vi "Module - RH_JONATHAN_LAMA.vi"() -> ()   [LabVIEW 2020]
uses:
  Control/State - eFGV.ctl
panel:
  out "Site Name":string="RH JONATHAN (13.65 kWp)"
  out "BANK-02-TEMP":dbl caption="T_bat" format="%#_g °C"
  out "BANK-02-IDC":dbl caption="I_bat" format="%#_g A"
  out "BANK-02-VDC":dbl caption="V_bat" format="%#_g V"
  out "BANK-02-SOC":dbl caption="SOC" format="%#_g %"
  out "PM-01-STATUS":bool
  out "SI-M-STATUS":bool
  out "BANK-01-TEMP":dbl caption="T_bat" format="%#_g °C"
  out "BANK-01-IDC":dbl caption="I_bat" format="%#_g A"
  out "BANK-01-VDC":dbl caption="V_bat" format="%#_g V"
  out "BANK-01-SOC":dbl caption="SOC" format="%#_g %"
  out "SB-02-STATUS":bool
  out "SB-02-B-IDC":dbl caption="B.Idc" format="%.0f A"
  out "SB-02-B-VDC":dbl caption="B.Vdc" format="%.0f V"
  out "SB-02-A-IDC":dbl caption="A.Idc" format="%.0f A"
  out "SB-02-A-VDC":dbl caption="A.Vdc" format="%.0f V"
  out "SB-02-PAC":dbl caption="Pac" format="%#_g W"
  out "SB-01-STATUS":bool
  out "SB-01-B-IDC":dbl caption="B.Idc" format="%.1f A"
  out "SB-01-B-VDC":dbl caption="B.Vdc" format="%.0f V"
  out "SB-01-A-IDC":dbl caption="A.Idc" format="%.1f A"
  out "SB-01-A-VDC":dbl caption="A.Vdc" format="%.0f V"
  out "SB-01-PAC":dbl caption="Pac" format="%.0f W"
  out "PM-01-FREQ":dbl caption="Freq" format="%.0f Hz"
  out "PM-01-IAC":dbl caption="Iac" format="%.0f A"
  out "PM-01-VAC":dbl caption="Vac" format="%.0f V"
  out "PM-01-PAC":dbl caption="Pac" format="%.0f W"
  out "SI-M-FREQ":dbl caption="FREQ" format="%.0f Hz"
  out "SI-M-L3":dbl caption="L3" format="%.0f V"
  out "SI-M-L2":dbl caption="L2" format="%.0f V"
  out "SI-M-L1":dbl caption="L1" format="%.0f V"
  out "SI-M-PAC":dbl caption="Pac" format="%.0f W"
  # "BANK-1"
  # "BANK-2"
  # "SI"
  # "PM-01"
  # "SB-02"
  # "SB-01"
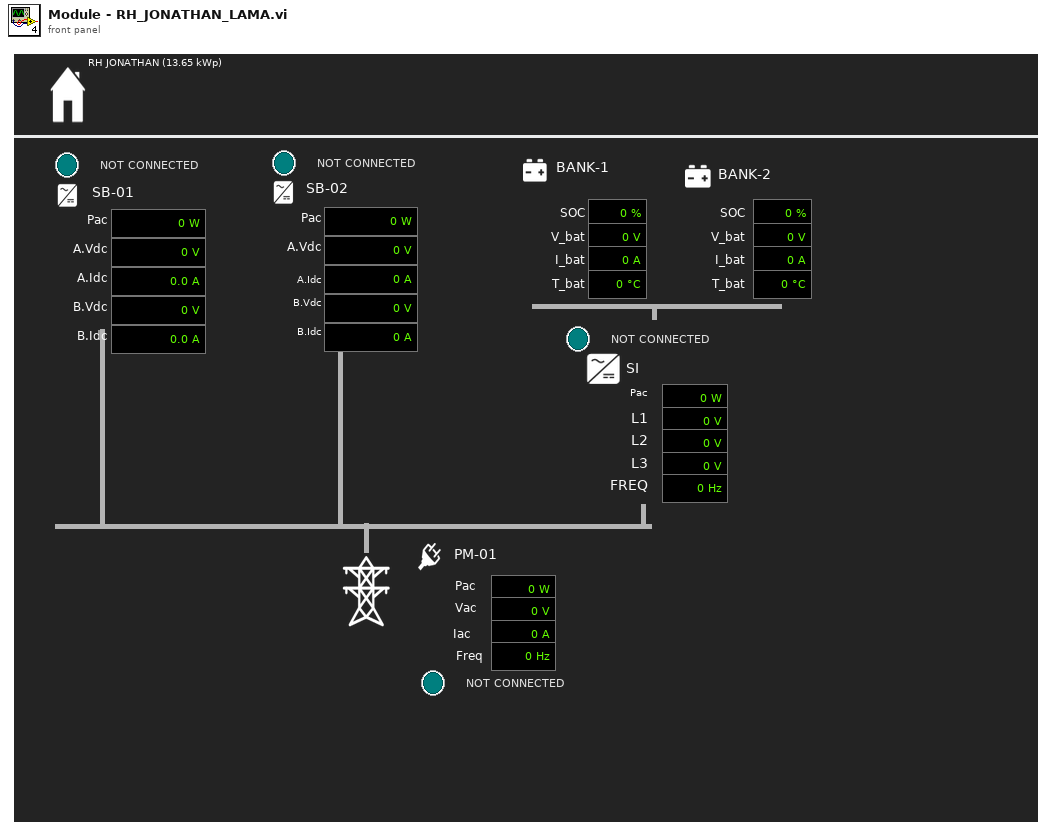
[diagram p1: front panel]
types:
  T1 = typedef "State - eFGV.ctl" = enum16{"Init", "Read", "Write", "Close"}
  T2 = typedef "Device Name.ctl" = enum16{"SB-01", "SB-02", "BANK-01", "BANK-02", "SI-M", "SI-S01", "SI-S02", "PM-01"}
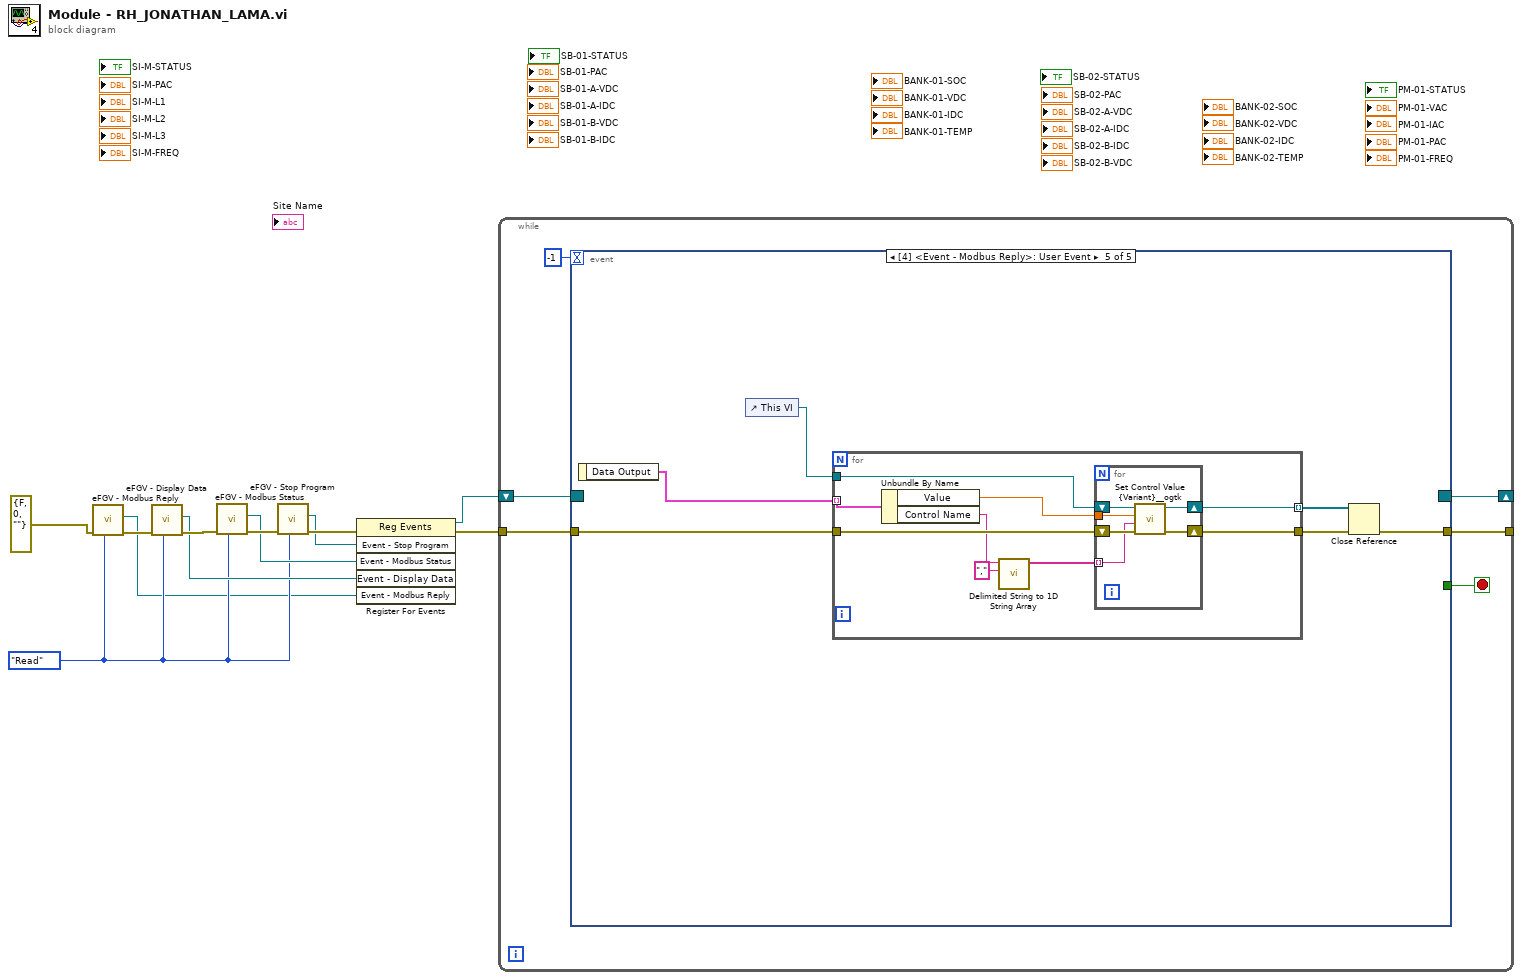
[diagram p0: block diagram]
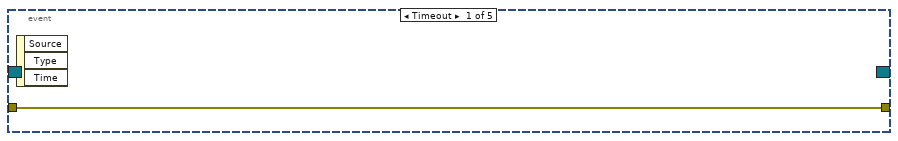
[diagram p2: hidden frame]
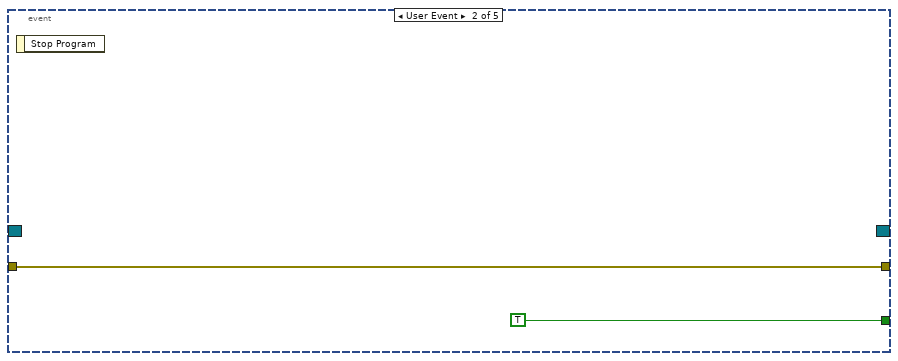
[diagram p3: hidden frame]
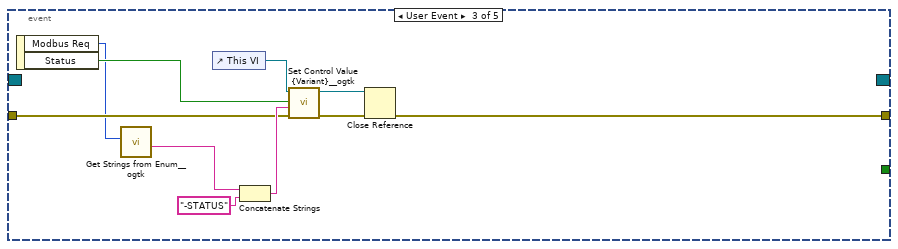
[diagram p4: hidden frame]
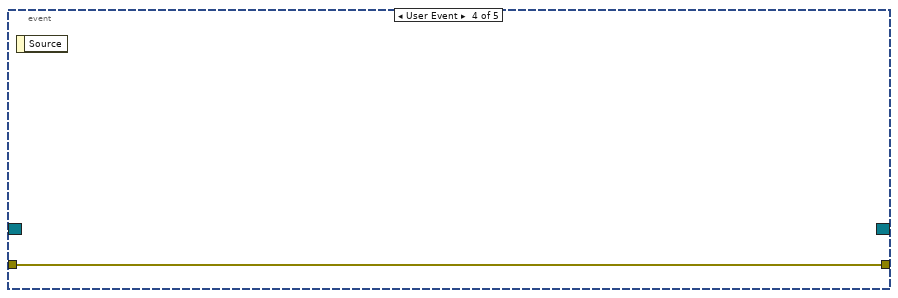
[diagram p5: hidden frame]
diagram:
  w2 = State_-_eFGV."Read" ("State - eFGV")
  n1 = call "eFGV - Modbus Reply.vi"("State - eFGV"=w2, "error in (no error)"=errorcluster {"status"=FALSE, "code"=0, "source"=""}) -> ("error out"=w4:errorcluster, "Event - Modbus Reply"=w1:refnum<user-event>)  [unwired: 8 in]
  n2 = call "eFGV - Display Data.vi"("State - eFGV"=w2, "error in (no error)"=w4) -> ("error out"=w6:errorcluster, "Event - Display Data"=w5:refnum<user-event>)  [unwired: 8 in]
  n3 = call "eFGV - Modbus Status.vi"("State - eFGV"=w2, "error in (no error)"=w6) -> ("error out"=w8:errorcluster, "Event - Modbus Status"=w7:refnum<user-event>)  [unwired: 8 in]
  n4 = call "eFGV - Stop Program.vi"("State - eFGV"=w2, "error in (no error)"=w8) -> ("error out"=w11:errorcluster, "Event - Stop Program"=w10:refnum<user-event>)  [unwired: 8 in]
  n5 = register-events(error in=w11, w10, w7, w5, w1) -> (reference out=w9:refnum<event-registration>, error out=w12:errorcluster)  [unwired: 1 in]
  n6 = while {
    tunnel: w12 -> [w17]
    shift-right: [w16] -> _
    shift-left: w9 -> [w18]
    tunnel: [w13] -> _
    stop <- w15 stop-if-true
    n7 = event shown="[4] <Event - Modbus Reply>: User Event" {
      selector: w18 -> [_ _ _ _ _]
      dyn-events: [_ _ _ _ _] -> w16
      timeout: -1 -> [_ _ _ _ _]
      tunnel: w17 -> [w19 w20 w29 w32 w37]
      tunnel: [_ TRUE _ _ _] -> w15
      tunnel: [w19 w20 w26 w32 w33] -> w13
      event Timeout {
        n8 = event-data() -> ()  [unwired: 1 in, 3 out]
      }
      event User Event {
        n9 = event-data() -> ()  [unwired: 1 in, 1 out]
      }
      event User Event {
        n10 = event-data() -> ("Modbus Req"=w24:T2, "Status"=w28:bool)  [unwired: 1 in]
        n11 = call <userlib>:"Get Strings from Enum__ogtk.vi"("Enum"=w24) -> ("String Value"=w23:string)  [unwired: 7 in, 3 out]
        n12 = control-ref of="This VI"() -> (w31:refnum<vi>)
        n13 = Concatenate Strings(w23, "-STATUS" ("string")) -> (w30:string)
        n14 = call <userlib>:"Set Control Value {Variant}__ogtk.vi"("error in (no error)"=w29, "Control Name (\"\": use variant name)"=w30, "Value"=w28, "VI Refnum"=w31) -> ("error out"=w27:errorcluster, "VI Refnum dup"=w25:refnum<vi>)  [unwired: 6 in]
        n15 = Close Reference(reference=w25, error in (no error)=w27) -> (error out=w26:errorcluster)
      }
      event User Event {
        n16 = event-data() -> ()  [unwired: 1 in, 1 out]
      }
      event User Event {
        n17 = event-data() -> ("Data Output"=w34:cluster{"Control Name":string, "Value":dbl}[])  [unwired: 1 in]
        n18 = control-ref of="This VI"() -> (w38:refnum<vi>)
        n19 = for {
          tunnel: w38 -> [w47]
          tunnel: w37 -> [w46]
          tunnel: [w45] -> w36
          tunnel: [w44] -> w35 mode=indexing
          tunnel: w34 -> [w43] mode=indexing
          n20 = Unbundle By Name(w43) -> ("Value"=w42:dbl, "Control Name"=w41:string)
          n21 = call <vilib>:"Delimited String to 1D String Array.vi"("delimiter"=",", "delimited string"=w41) -> ("string array"=w39:string[])  [unwired: 9 in]
          n22 = for {
            tunnel: w42 -> [w49]
            shift-right: [w50] -> w44
            shift-left: w47 -> [w53]
            shift-right: [w51] -> w45
            shift-left: w46 -> [w52]
            tunnel: w39 -> [w48] mode=indexing
            n23 = call <userlib>:"Set Control Value {Variant}__ogtk.vi"("error in (no error)"=w52, "Control Name (\"\": use variant name)"=w48, "Value"=w49, "VI Refnum"=w53) -> ("error out"=w51:errorcluster, "VI Refnum dup"=w50:refnum<vi>)  [unwired: 6 in]
          }
        }
        n24 = Close Reference(reference=w35, error in (no error)=w36) -> (error out=w33:errorcluster)
      }
    }
  }
